vi "get_version_numbers.vi"(8 "error in (no error)":errorcluster, 11 "VISA resource name":refnum<visa-resource-name>) -> (0 "error out":errorcluster, 2 "Version numbers":T1, 3 "VISA resource name out":refnum<visa-resource-name>)   [LabVIEW 2018, in "Inficon IC6.lvlib"]
doc: "Query structure, compatibility, and range version numbers."
uses:
  <instrlib>/Inficon IC6/Inficon IC6.lvlib
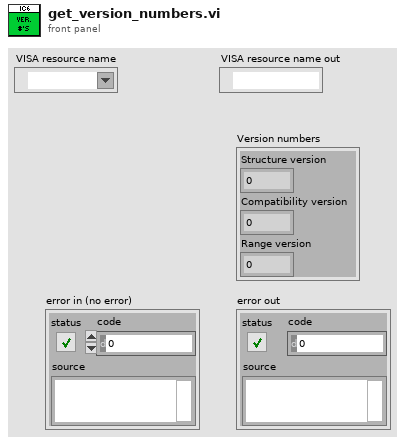
[diagram p1: front panel]
types:
  T1 = cluster{"Structure version":i32, "Compatibility version":i32, "Range version":i32}
  T2 = enum16{"Source", "General", "Input name", "Process name", "Logic", "Material", "Material name", "Output name", "Process", "Sensor", "Output type", "User message", "Layer", ""}
  T3 = enum16{"Hello", "Query", "Remote action", "Status", "Update"}
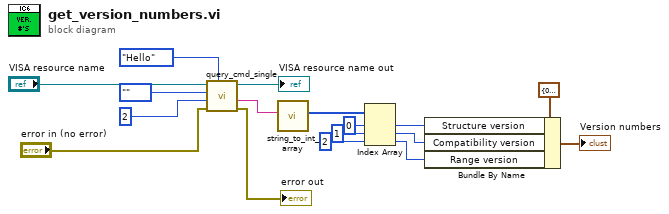
[diagram p0: block diagram]
diagram:
  n1 = call <instrlib>:"query_cmd_single.vi"("Command group"=T3."Hello", "error in (no error)"="error in (no error)", "Command ID"=u8 2, "Command subgroup"=T2."", "VISA resource name"="VISA resource name") -> ("error out"=→"error out":errorcluster, "formatted response"=w11:string, "VISA resource name out"=→"VISA resource name out":refnum<visa-resource-name>)  [unwired: 2 in, 2 out]
  n2 = call <instrlib>:"string_to_int_array.vi"("Ints"=w11) -> ("Int array"=w10:i32[])  [unwired: 9 in, 1 out]
  n3 = Index Array(array=w10, index #1=0 ("index"), index #2=1 ("index"), index #3=2 ("index")) -> (element #1=w5:i32, element #2=w4:i32, element #3=w3:i32)
  n4 = Bundle By Name(cluster=T1 {"Structure version"=0, "Compatibility version"=0, "Range version"=0} ("input cluster"), "Structure version"=w5, "Compatibility version"=w4, "Range version"=w3) -> (→"Version numbers":T1)
